vi "Read Elevator Positions from Config.vi"(8 "error in (no error)":errorcluster, 11 "Settings":variant) -> (0 "error out":errorcluster, 2 "Arm Positions":T1, 3 "Settings out":variant)   [LabVIEW 2019, in "Elevator.lvlib" / "Elevator.lvclass"]
doc: "This VI reads the elevator positions from the configuration file and loads them into the type def."
uses:
  Elevator.lvclass
  Controls/Arm Position Values.ctl
  f974b54b-b998-412c-9bf9-c72a43652bb5.vi
  <vilib>/Utility/error.llb/Trim Whitespace.vi
  <vilib>/Utility/error.llb/Error Cluster From Error Code.vi
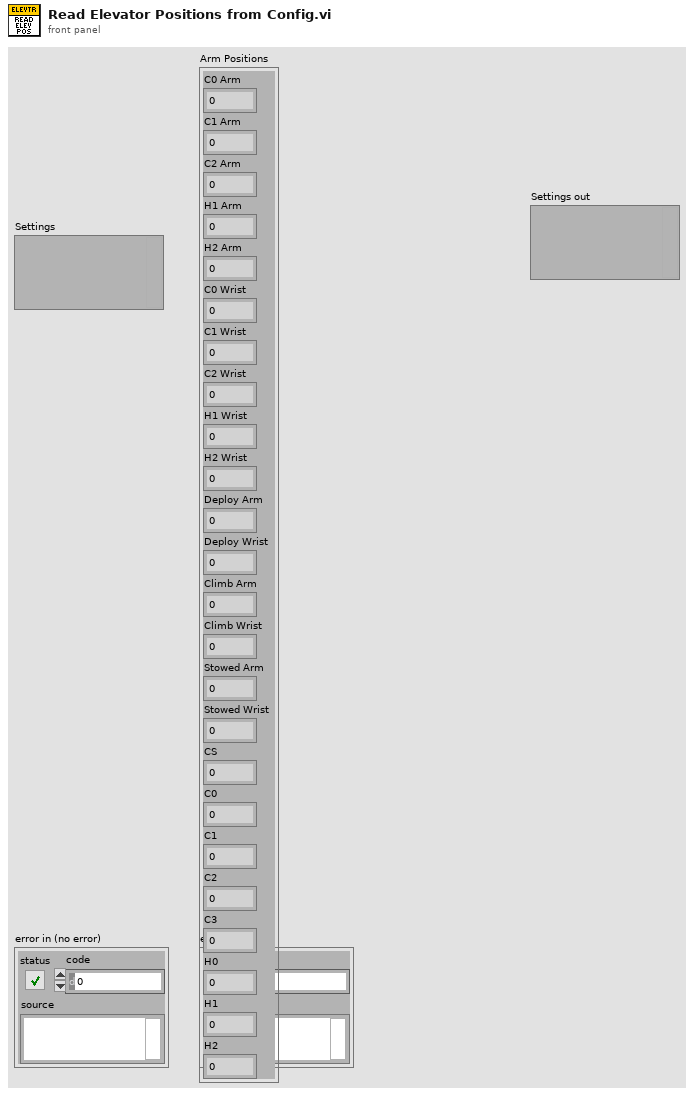
[diagram p1: front panel]
types:
  T1 = typedef "Elevator.lvlib/Elevator.lvclass/Arm Position Values.ctl" = cluster{"C0 Arm":dbl, "C1 Arm":dbl, "C2 Arm":dbl, "H1 Arm":dbl, "H2 Arm":dbl, "C0 Wrist":dbl, "C1 Wrist ":dbl, "C2 Wrist":dbl, "H1 Wrist":dbl, "H2 Wrist":dbl, "Deploy Arm":dbl, "Deploy Wrist":dbl, "Climb Arm":dbl, "Climb Wrist":dbl, "Stowed Arm":dbl, "Stowed Wrist":dbl, "CS":dbl, "C0":dbl, "C1":dbl, "C2":dbl, "C3":dbl, "H0":dbl, "H1":dbl, "H2":dbl}
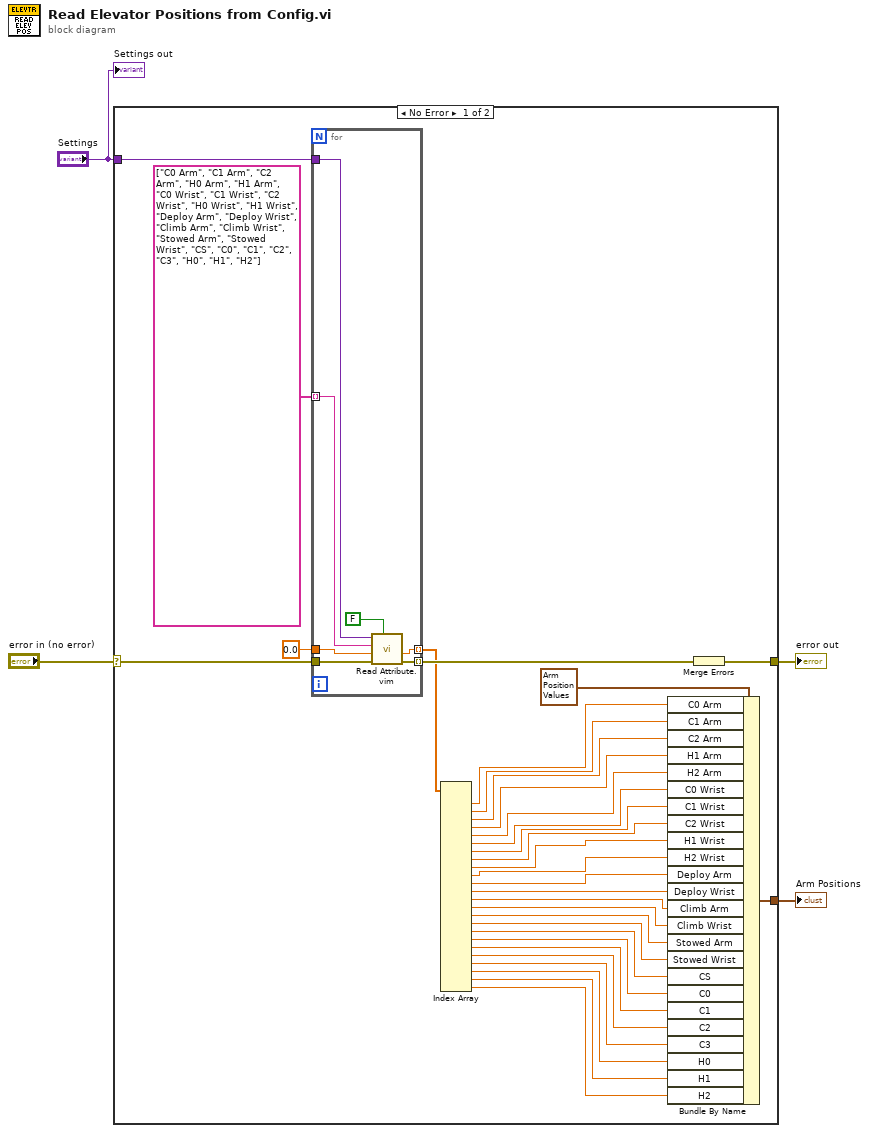
[diagram p0: block diagram]
diagram:
  n1 = case shown="No Error" "error in (no error)" {
    selector: "error in (no error)" -> [w31 w45]
    tunnel: [w37 w45] -> w4
    tunnel: [w35 _] -> w3
    tunnel: "Settings" -> [w30 _]
    frame No Error {
      n2 = for {
        tunnel: w30 -> [w44]
        tunnel: w31 -> [w43]
        tunnel: string[] ["C0 Arm", "C1 Arm", "C2 Arm", "H0 Arm", "H1 Arm", "C0 Wrist", "C1 Wrist", "C2 Wrist", "H0 Wrist", "H1 Wrist", "Deploy Arm", "Deploy Wrist", "Climb Arm", "Climb Wrist", "Stowed Arm", "Stowed Wrist", "CS", "C0", "C1", "C2", "C3", "H0", "H1", "H2"] ("keys") -> [w42] mode=indexing
        tunnel: 0.0 ("C0 Arm") -> [w41]
        tunnel: [w40] -> w29 mode=indexing
        tunnel: [w39] -> w36 mode=indexing
        n3 = call "Read Attribute.vim"("Error if not found (T)"=FALSE, "error in"=w43, "default value (data type)"=w41, "name"=w42, "variant in"=w44) -> ("error out"=w39:errorcluster, "value"=w40:dbl)  [unwired: 3 in, 2 out]
      }
      n4 = Index Array(array=w29) -> (element #1=w28:dbl, element #2=w27:dbl, element #3=w26:dbl, element #4=w25:dbl, element #5=w24:dbl, element #6=w23:dbl, element #7=w22:dbl, element #8=w21:dbl, element #9=w20:dbl, element #10=w19:dbl, element #11=w18:dbl, element #12=w17:dbl, element #13=w16:dbl, element #14=w15:dbl, element #15=w14:dbl, element #16=w13:dbl, element #17=w12:dbl, element #18=w11:dbl, element #19=w10:dbl, element #20=w9:dbl, element #21=w8:dbl, element #22=w7:dbl, element #23=w6:dbl, element #24=w5:dbl)  [unwired: 24 in]
      n5 = Bundle By Name(cluster=T1 {"C0 Arm"=0.0, "C1 Arm"=0.0, "C2 Arm"=0.0, "H1 Arm"=0.0, "H2 Arm"=0.0, "C0 Wrist"=0.0, "C1 Wrist "=0.0, "C2 Wrist"=0.0, "H1 Wrist"=0.0, "H2 Wrist"=0.0, "Deploy Arm"=0.0, "Deploy Wrist"=0.0, "Climb Arm"=0.0, "Climb Wrist"=0.0, "Stowed Arm"=0.0, "Stowed Wrist"=0.0, "CS"=0.0, "C0"=0.0, "C1"=0.0, "C2"=0.0, "C3"=0.0, "H0"=0.0, "H1"=0.0, "H2"=0.0} ("Arm Positions"), "C0 Arm"=w28, "C1 Arm"=w27, "C2 Arm"=w26, "H1 Arm"=w25, "H2 Arm"=w24, "C0 Wrist"=w23, "C1 Wrist"=w22, "C2 Wrist"=w21, "H1 Wrist"=w20, "H2 Wrist"=w19, "Deploy Arm"=w18, "Deploy Wrist"=w17, "Climb Arm"=w16, "Climb Wrist"=w15, "Stowed Arm"=w14, "Stowed Wrist"=w13, "CS"=w12, "C0"=w11, "C1"=w10, "C2"=w9, "C3"=w8, "H0"=w7, "H1"=w6, "H2"=w5) -> (w35:T1)
      n6 = Merge Errors(w36) -> (w37:errorcluster)
    }
    frame Error {
    }
  }
  "error out" <- w4
  "Arm Positions" <- w3
  "Settings out" <- "Settings"
